vi "Read DAQ Type.vi"(8 "error in (no error)":errorcluster, 11 "PXIe 2737 in":refnum<class "PXIe 2737.lvclass">) -> (0 "error out":errorcluster, 2 "DAQ Type":enum16{"Hardware", "Simulation"}(ring), 3 "PXIe 2737 out":refnum<class "PXIe 2737.lvclass">)   [LabVIEW 2021, in "S-Matrix.lvlib" / "PXIe 2737.lvclass"]
uses:
  PXIe 2737.lvclass
  PXIe 2737.lvclass/PXIe 2737.ctl
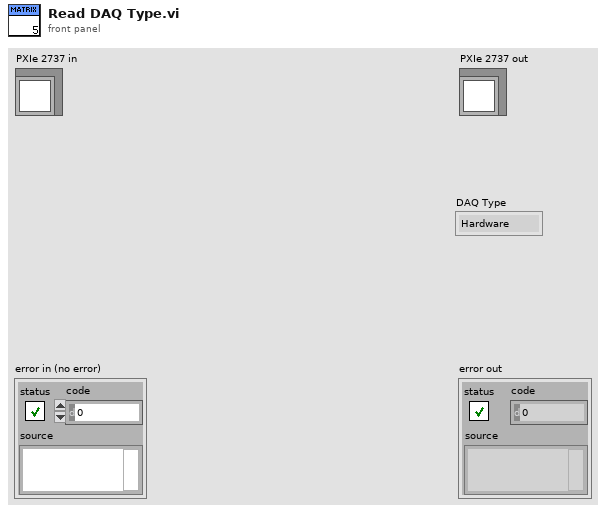
[diagram p1: front panel]
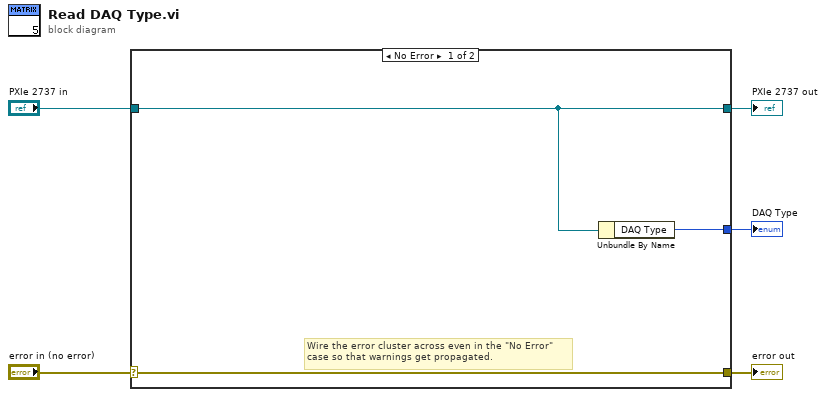
[diagram p0: block diagram]
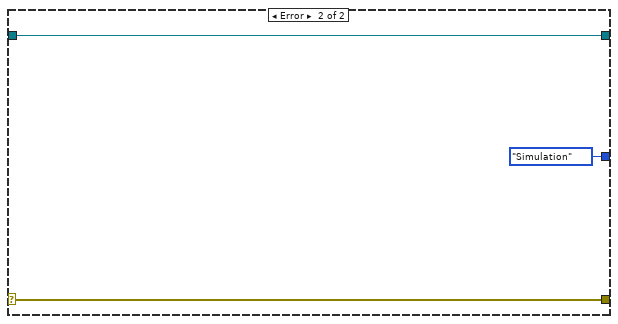
[diagram p2: hidden frame]
diagram:
  n1 = case shown="No Error" "error in (no error)" {
    selector: "error in (no error)" -> [w8 w11]
    tunnel: [w8 w11] -> w4
    tunnel: [w7 w10] -> w2
    tunnel: "PXIe 2737 in" -> [w7 w10]
    tunnel: [w6 enum16{"Hardware", "Simulation"}."Simulation" ("DAQ Type")] -> w1
    frame No Error {
      # "Wire the error cluster across even in the \"No Error\"\ncase so that warnings get propagated."
      n2 = Unbundle By Name(w7) -> ("DAQ Type"=w6:enum16{"Hardware", "Simulation"})
    }
    frame Error {
    }
  }
  "error out" <- w4
  "PXIe 2737 out" <- w2
  "DAQ Type" <- w1
